vi "Subpanel - Coercion Test.vi"(0 "VI Reference In":refnum<vi>, 5 "Subpanel Details":string, 11 "error in (no error)":errorcluster) -> (4 "VI Reference Out":refnum<vi>, 15 "error out":errorcluster)   [LabVIEW 2016]
uses:
  apis/Stimulus/KeyBoardSimulation/Core/KeyBoardSimulation.vi
  apis/Assert/AssertControlValue/Equal.vi
  <vilib>/addons/_JKI Toolkits/Caraya/classes/Test/Test.lvclass
  Drona.lvlib
  apis/Stimulus/KeyBoardSimulation/KeyboardSimulation.lvlib
  apis/Assert/AssertControlValue/AssertControlValue.lvlib
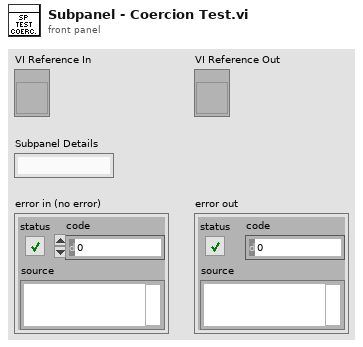
[diagram p1: front panel]
types:
  T1 = cluster{"Test Label":string, "Key In Array":cluster{" Key":u8, "Action":enum16{"Press", "Up", "Down"}, "Delay (ms)":u32}[], "Assert Value":dbl}[]
  T2 = cluster{" Key":u8, "Action":enum16{"Press", "Up", "Down"}, "Delay (ms)":u32}[]
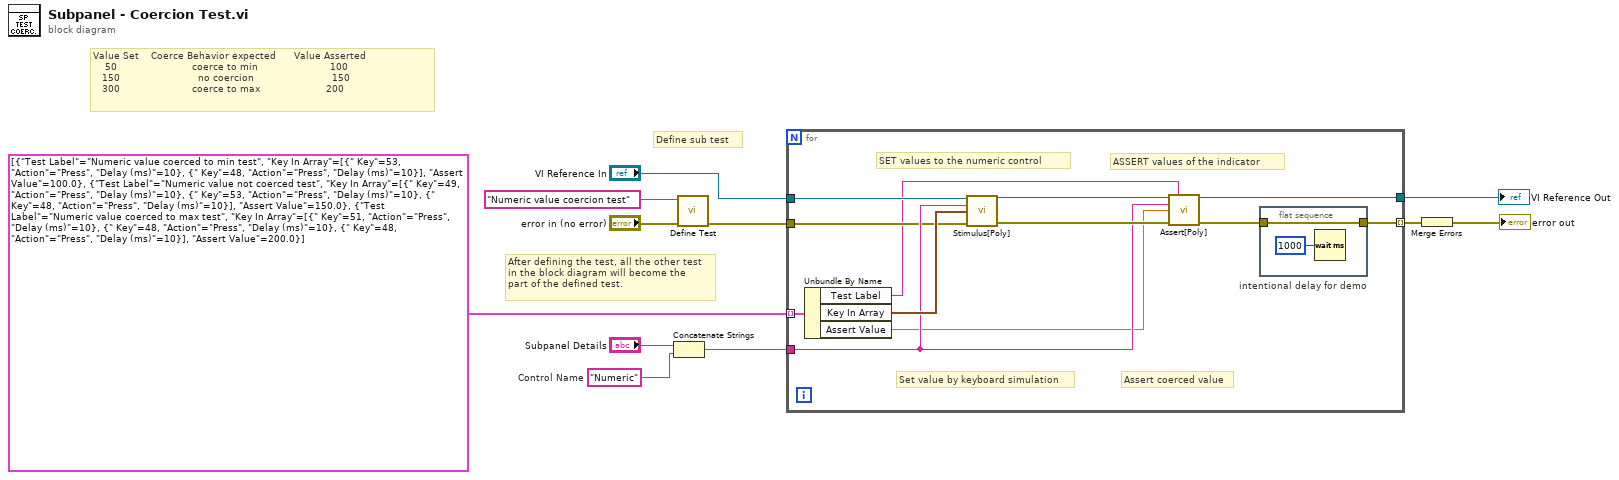
[diagram p0: block diagram]
diagram:
  w8 = "Numeric"  # Control Name
  # "Value Set    Coerce Behavior expected      Value Asserted\n    50                         coerce to min                        100\n   150                          no coercion                          150\n   300                        coerce to max                      200"
  # "After defining the test, all the other test\nin the block diagram will become the \npart of the defined test."
  # "Define sub test"
  n1 = Concatenate Strings("Subpanel Details", w8) -> (w7:string)
  n2 = call <vilib>:"Define Test.vi"("error in (no error)"="error in (no error)", "Label (VI Title)"="Numeric value coercion test") -> ("error out"=w3:errorcluster)  [unwired: 9 in]
  n3 = for {
    tunnel: T1 [{"Test Label"="Numeric value coerced to min test", "Key In Array"=[{" Key"=53, "Action"=enum."Press", "Delay (ms)"=10}, {" Key"=48, "Action"=enum."Press", "Delay (ms)"=10}], "Assert Value"=100.0}, {"Test Label"="Numeric value not coerced test", "Key In Array"=[{" Key"=49, "Action"=enum."Press", "Delay (ms)"=10}, {" Key"=53, "Action"=enum."Press", "Delay (ms)"=10}, {" Key"=48, "Action"=enum."Press", "Delay (ms)"=10}], "Assert Value"=150.0}, {"Test Label"="Numeric value coerced to max test", "Key In Array"=[{" Key"=51, "Action"=enum."Press", "Delay (ms)"=10}, {" Key"=48, "Action"=enum."Press", "Delay (ms)"=10}, {" Key"=48, "Action"=enum."Press", "Delay (ms)"=10}], "Assert Value"=200.0}] -> [w23] mode=indexing
    tunnel: w7 -> [w19]
    tunnel: "VI Reference In" -> [w18]
    tunnel: w3 -> [w17]
    tunnel: [w15] -> w4 mode=indexing
    tunnel: [w12] -> w2
    # "Set value by keyboard simulation"
    # "Assert coerced value"
    # "ASSERT values of the indicator"
    # "SET values to the numeric control"
    n4 = Unbundle By Name(w23) -> ("Test Label"=w13:string, "Key In Array"=w20:T2, "Assert Value"=w14:dbl)
    n5 = call-poly "Stimulus[Poly].vi"("VI Reference In"=w18, "Control Path"=w19, "Key Array"=w20, "error In"=w17) -> ("VI Reference Out"=w21:refnum<vi>, "error IO"=w22:errorcluster)  [unwired: 10 in]
    n6 = call-poly "Assert[Poly].vi"("VI Reference In"=w21, "Label"=w13, "Control Path"=w19, "Control Value"=w14, "Error In"=w22) -> ("VI Reference Out"=w12:refnum<vi>, "Error Out"=w16:errorcluster)  [unwired: 9 in]
    n7 = flat-sequence "intentional delay for demo" {
      tunnel: w16 -> [w24]
      tunnel: [w24] -> w15
      frame #0 {
        n8 = Wait (ms)(milliseconds to wait=u32 1000) -> ()  [unwired: 1 out]
      }
    }
  }
  "VI Reference Out" <- w2
  n9 = Merge Errors(w4) -> (→"error out":errorcluster)
